vi "UHR-Fleezers Control (host) - 10.7.vi"() -> ()   [LabVIEW 2011] (continued)
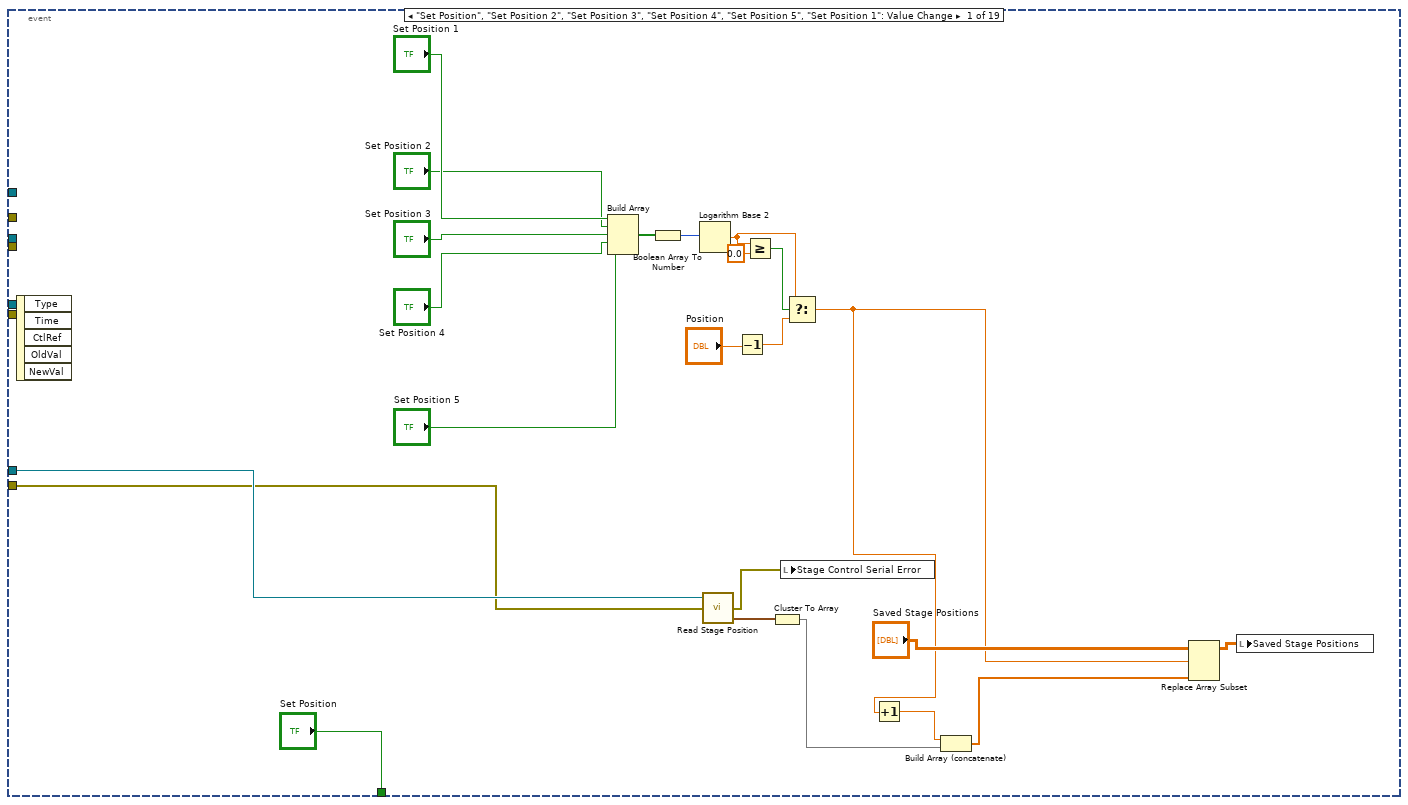
[diagram p2: hidden frame]
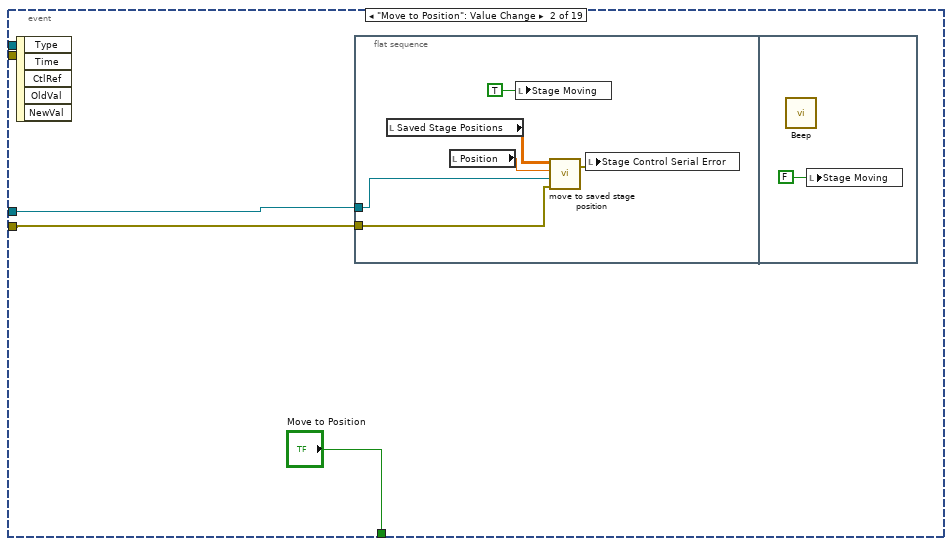
[diagram p3: hidden frame]
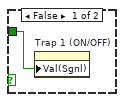
[diagram p5: hidden frame]
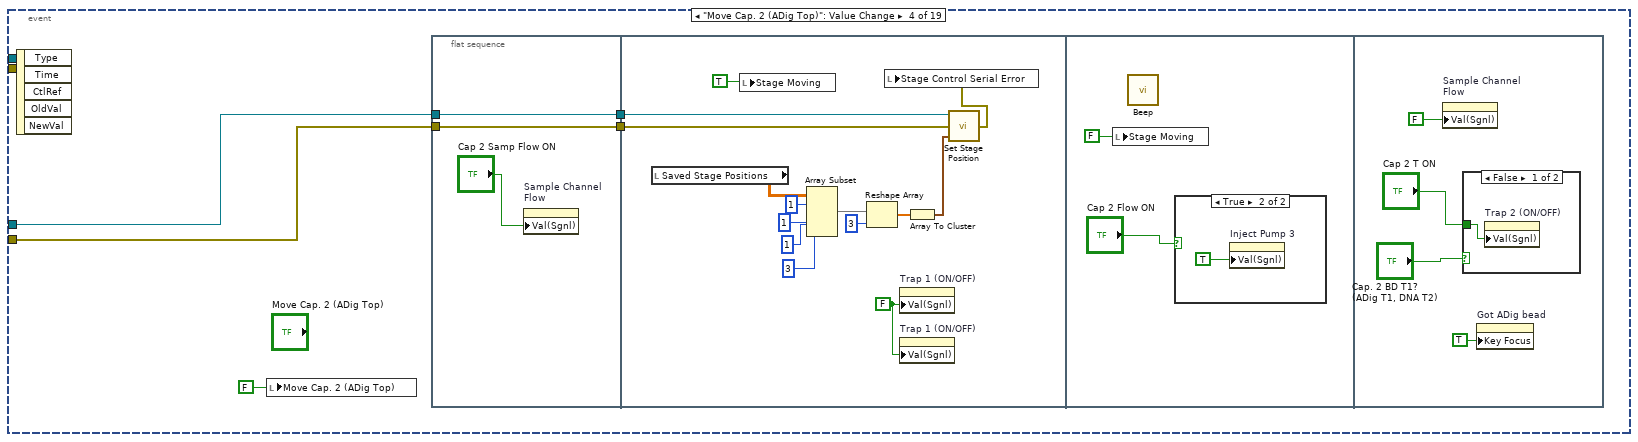
[diagram p6: hidden frame]
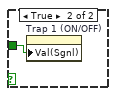
[diagram p8: hidden frame]
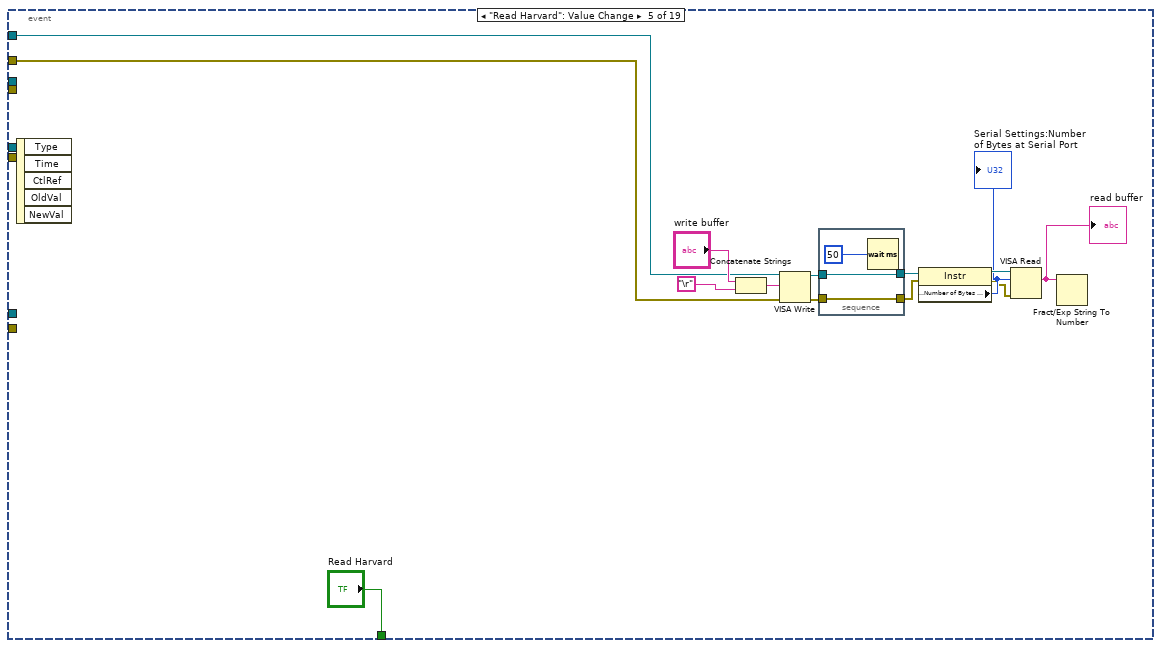
[diagram p9: hidden frame]
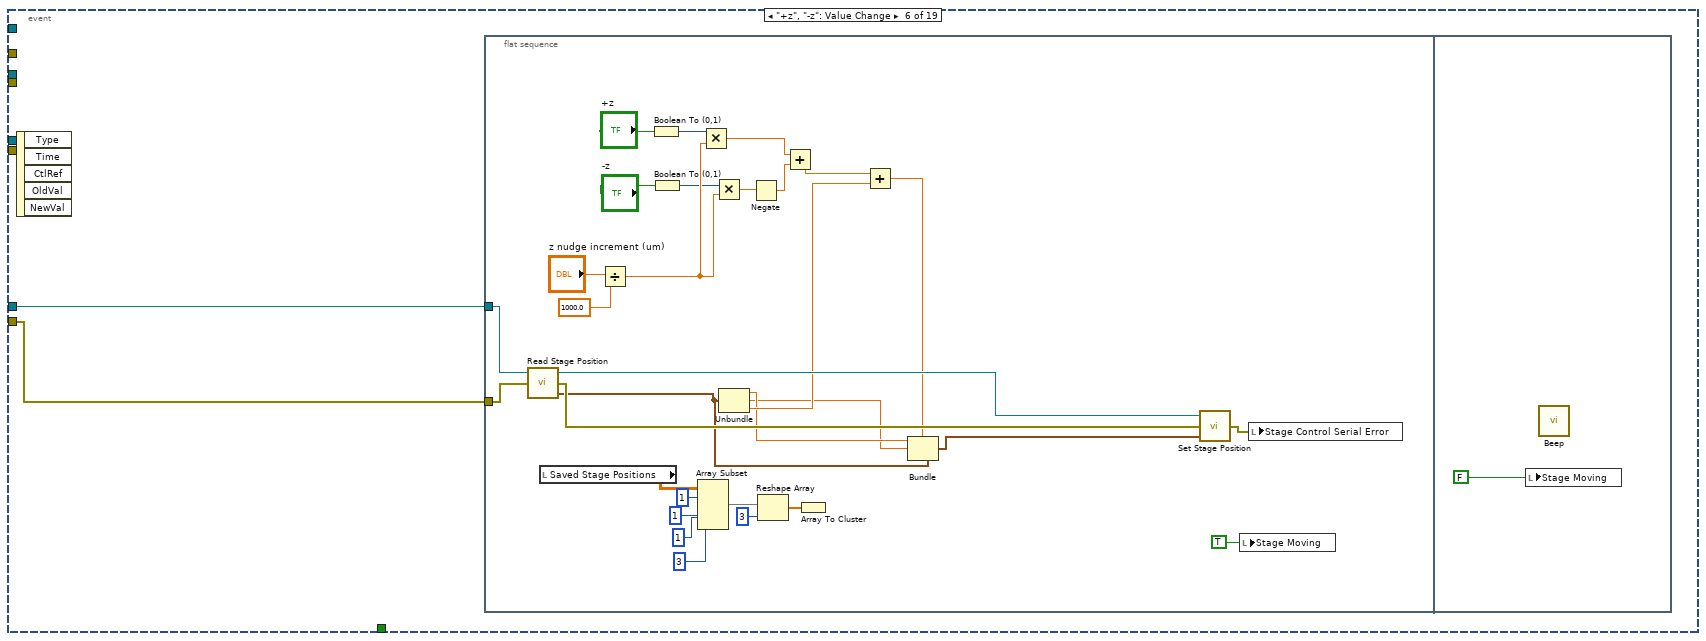
[diagram p10: hidden frame]
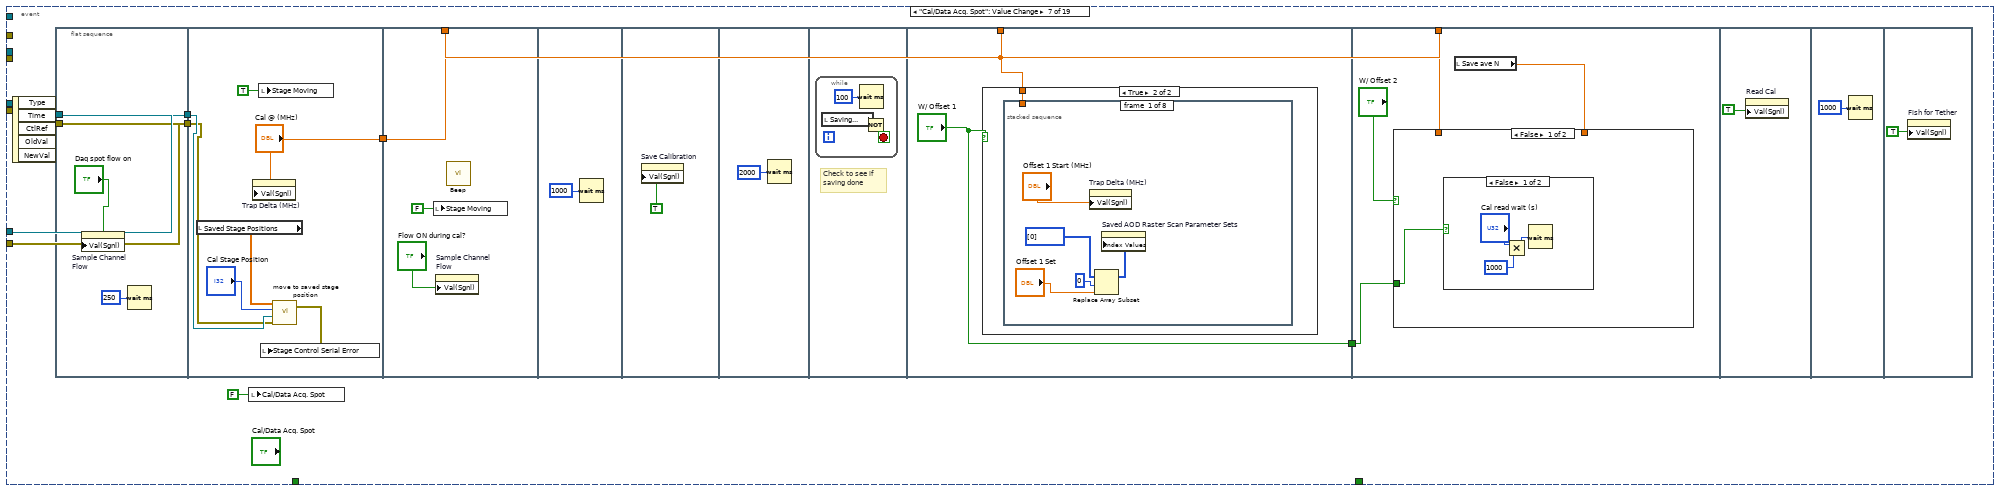
[diagram p11: hidden frame]
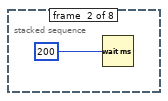
[diagram p13: hidden frame]
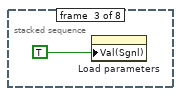
[diagram p14: hidden frame]
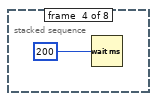
[diagram p15: hidden frame]
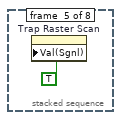
[diagram p16: hidden frame]
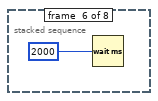
[diagram p17: hidden frame]
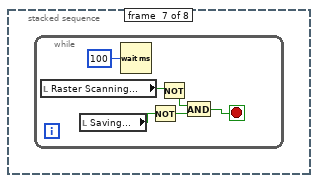
[diagram p18: hidden frame]
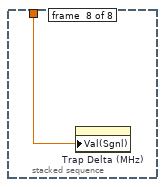
[diagram p19: hidden frame]
                n2754 = call <vilib>:"Mean.vi"("X"=w4456) -> ("mean"=w4449:dbl)  [unwired: 1 out]
                n2755 = Subtract(x=w4450, y=w4449) -> (x-y=w4440:dbl)
                "Delta Fl. 2" <- w4440
                n2756 = Subtract(x=w4475, y=w4474) -> (x-y=w4472:dbl)
                "Delta Fl. 1" <- w4472
                n2757 = Initialize Array(w4472, 1 ("dimension size")) -> (w4469:dbl[])
                n2758 = Initialize Array(w4440, 1 ("dimension size")) -> (w4446:dbl[])
                n2759 = feedback #38(w4469) -> (w4470:dbl[])
                n2760 = Build Array (concatenate)(w4470, w4469) -> (w4468:dbl[])
                n2761 = feedback #39(w4446) -> (w4447:dbl[])
                n2762 = Build Array (concatenate)(w4447, w4446) -> (w4445:dbl[])
                n2763 = Select(t=w4469, s=w4441, f=w4468) -> (s? t:f=w4444:dbl[])
                n2764 = feedback-in #38(w4444) -> ()
                n2765 = Select(t=w4446, s=w4441, f=w4445) -> (s? t:f=w4443:dbl[])
                n2766 = feedback-in #39(w4443) -> ()
                n2767 = Build Array(w4444, w4443) -> (→"Save APD Deriv":dbl[][])
              }
            }
            "Progress" <- w4417
            "Progress 2" <- w4417
          }
        }
      }
    }
    n2768 = Bundle By Name(cluster=w3079, "Green FB Ch 0"=w3078, "Green FB Ch 1"=w3077) -> (w3057:T47)
    "Green FB Signals (V)" <- w3057
    n2769 = Unbundle By Name(w3057) -> ("Green FB Ch 2"=→"Green FB Plot":dbl)
    n2770 = local read "wait to reset values"() -> (w3148:bool)
    n2771 = Not(x=w3146) -> (.not. x?=w3149:bool)
    n2772 = And(x=w3149, y=w3148) -> (x .and. y?=w3150:bool)
    n2773 = case "Part of MCL raster scanning: returns to initial positions after scan done" shown="True" w3150 {
      tunnel: w2863 -> [w3959 w3966]
      tunnel: [w3959 w3965] -> w3152
      tunnel: w2862 -> [w3958 w3964]
      tunnel: [w3958 w3963] -> w3147
      frame False {
      }
      frame True {
        w3974 = 10.0 ("y")
        w3973 = 32767.0 ("y")
        # "to return scan values\nafter a synchronous \nAOM scan"
        n2774 = local read "AO2"() -> (w3967:dbl)
        n2775 = local read "AO1"() -> (w3968:dbl)
        n2776 = local write "wait to reset values"(FALSE ("wait to reset values")) -> ()
        n2777 = Multiply(x=w3968, y=w3973) -> (x*y=w3970:dbl)
        n2778 = Multiply(x=w3967, y=w3973) -> (x*y=w3972:dbl)
        n2779 = Divide(x=w3970, y=w3974) -> (x/y=w3969:dbl)
        n2780 = Divide(x=w3972, y=w3974) -> (x/y=w3971:dbl)
        n2781 = To Word Integer(number=w3969) -> (16bit integer=w3975:i16)
        n2782 = To Word Integer(number=w3971) -> (16bit integer=w3976:i16)
        n2783 = local read "Total Counts (ticks)"() -> (w3960:u32)
        n2784 = xnode "Read/Write Control"("FPGA VI Reference In"=w3966, "error in"=w3964, "AO1"=w3975, "AO2"=w3976, "MCL count"=w3960) -> ("FPGA VI Reference Out"=w3965:T19, "error out"=w3963:errorcluster)
        n2785 = local read "Scan Range (V)\n(of steps)"() -> (w3961:dbl)
        n2786 = property on="Scan Range (V)\n(of steps)" class="DigNum (strict)"("Val(Sgnl)"=w3961) -> ()  [unwired: 2 in, 2 out]
      }
    }
    n2787 = node-c288() -> ()  [unwired: 2 out]
  }
  n2788 = node-c288(w91) -> ()  [unwired: 1 out]
  n2789 = node-c288(w93) -> ()  [unwired: 1 out]
  n2790 = node-c288(w78) -> ()  [unwired: 1 out]
  n2791 = VISA Close(VISA resource name=w82, error in (no error)=w81) -> (error out=w130:errorcluster)
  n2792 = call <vilib>:"Simple Error Handler.vi"("error in (no error)"=w130) -> ()  [unwired: 1 in, 8 out]
  n2793 = node-c288(w89) -> ()  [unwired: 1 out]
  n2794 = node-c288(w174) -> ()  [unwired: 1 out]
  n2795 = flat-sequence {
    tunnel: w268 -> [w4547]
    tunnel: w270 -> [w4548]
    tunnel: [w4546] -> w249
    tunnel: [w4545] -> w248
    tunnel: w230 -> [_]
    tunnel: w182 -> [_]
    tunnel: w95 -> [_]
    tunnel: w249 -> [w4549]
    tunnel: w248 -> [w4550]
    frame #0 {
      w4544 = FALSE ("AI to FIFO")
      n2796 = xnode "Read/Write Control"("FPGA VI Reference In"=w4548, "error in"=w4547, "AI to FIFO"=w4544, "APD to FIFO"=w4544) -> ("FPGA VI Reference Out"=w4546:T19, "error out"=w4545:errorcluster)
    }
    frame #1 {
      n2797 = xnode "Close FPGA VI Reference"("FPGA VI Reference In"=w4549, "error in"=w4550) -> ("error out"=→"error out":errorcluster)
    }
  }
